vi "MainV1.vi"() -> ()   [LabVIEW 2019]
uses:
  <vilib>/userDefined/High Color/IMAQdx.ctl
  <vilib>/FPGAPlugInAG/myRIO-1900/niLvFpga_Open_myRIO-1900.vi
  <vilib>/rvi/interface/common/dynamic/niFpgaDynamicAddResources.vi
  <vilib>/Utility/error.llb/Error Cluster From Error Code.vi
  <vilib>/rvi/errors/niLvFpgaAdjustHostInterfaceError.vi
  <vilib>/FPGAPlugInAG/Dynamic/niLvFpga_Close_Dynamic.vi
  <vilib>/rvi/interface/nirviOpenFPGA/nirviOpenFPGA.xnode
  FPGA Bitfiles/MRmecanum_FPGATarget_FPGAMainModified_TerasRobot_LKSN2021.lvbitx
  <vilib>/rvi/interface/nirviReadWriteControl/nirviReadWriteControl.xnode
  <vilib>/rvi/interface/nirviCloseFPGA/nirviCloseFPGA.xnode
  NiFpgaLv.dll
  <vilib>/rvi/interface/Simulation/niFpgaSimulationCallBeginRW.vi
  <vilib>/vision/driver/NI_Vision_Acquisition_Software.lvlib
  <vilib>/vision/NI_Vision_Development_Module.lvlib
panel:
  out "Color Put":T1(plugin-control)
  in  "SERVO 3":u16
  in  "Value diatas brp?":u16
  in  "Value Udah ambil brp?":u16
  in  "M5  DOWN TIMES GRAB":u32=1
  in  "Udah ambil brp?":u16
  in  "Standcube diatas brp?":u16
  out "WHITE":bool
  out "TOXIC":bool
  out "BLUE":bool
  out "STOP ? 11":bool
  out "STOP ? 10":bool
  out "STOP ? 9":bool
  out "STOP ? 8":bool
  out "M5 up":i16=1000
  out "STOP ? 7":bool
  out "STOP ? 6":bool
  out "STOP ? 5":bool
  out "STOP ? 4":bool
  out "STOP ? 3":bool
  out "AND green":bool
  out "AND red":bool
  out "Red True":bool
  out "Green True":bool
  out "Locate Put":string
  out "Green Stand":bool
  out "Red Stand":bool
  out "STOP Open Grab":bool
  out "total":i16
  out "Index ke?":i32
  out "White Cube":bool
  out "Blue Cube":bool
  out "Toxic Cube":bool
  out "Color Grab":T1(plugin-control)
  in  "Color Sensitivity":u32(ring) items=["Low", "Medium", "High"]
  in  "Exposure Config Value":i64=10
  out "size(s)":i32
  in  "Session In":T2="cam1"
  out "Qrcode image":T1(plugin-control)
  out "Found ?":bool
  in  "Tab Control":T3(tab)
  in  "Main":T4(array[cluster])=[{"Time"=0.0, "Mode"=enum."Balance", "Speed"=250.0, "Gerakan"=enum."Maju"}, {"Time"=0.0, "Mode"=enum."Line Follow", "Speed"=150.0, "Gerakan"=enum."Kanan"}, {"Time"=0.0, "Mode"=enum."Qrcode", "Speed"=0.0, "Gerakan"=enum."Camera"}, {"Time"=1000.0, "Mode"=enum."Standard", "Speed"=100.0, "Gerakan"=enum."Mundur"}, {"Time"=3000.0, "Mode"=enum."Standard", "Speed"=300.0, "Gerakan"=enum."Kiri"}, {"Time"=0.0, "Mode"=enum."Balance", "Speed"=300.0, "Gerakan"=enum."Maju"}, {"Time"=2000.0, "Mode"=enum."Standard", "Speed"=815.0, "Gerakan"=enum."Putar Kiri"}, {"Time"=1300.0, "Mode"=enum."Standard", "Speed"=300.0, "Gerakan"=enum."Maju"}, {"Time"=0.0, "Mode"=enum."Balance", "Speed"=300.0, "Gerakan"=enum."Kanan"}, {"Time"=2100.0, "Mode"=enum."Standard", "Speed"=300.0, "Gerakan"=enum."Kiri"}]
  in  "Nurse":T4(array[cluster])=[{"Time"=2.0, "Mode"=enum."Standard", "Speed"=815.0, "Gerakan"=enum."Putar Kiri"}, {"Time"=0.0, "Mode"=enum."Balance", "Speed"=150.0, "Gerakan"=enum."Kiri"}, {"Time"=4.0, "Mode"=enum."Standard", "Speed"=300.0, "Gerakan"=enum."Maju"}, {"Time"=0.0, "Mode"=enum."Balance", "Speed"=150.0, "Gerakan"=enum."Kiri"}, {"Time"=0.0, "Mode"=enum."Line Follow", "Speed"=150.0, "Gerakan"=enum."Kanan"}, {"Time"=0.0, "Mode"=enum."Color Grab", "Speed"=0.0, "Gerakan"=enum."Camera"}, {"Time"=0.0, "Mode"=enum."Line Follow", "Speed"=200.0, "Gerakan"=enum."Kanan"}, {"Time"=0.0, "Mode"=enum."Color Put", "Speed"=0.0, "Gerakan"=enum."Camera"}]
  in  "Room 1":T4(array[cluster])
  in  "Room 2":T4(array[cluster])
  in  "Output":T4(array[cluster])=[{"Time"=0.0, "Mode"=enum."Balance", "Speed"=150.0, "Gerakan"=enum."Mundur"}, {"Time"=0.0, "Mode"=enum."Balance", "Speed"=150.0, "Gerakan"=enum."Kiri"}, {"Time"=5.0, "Mode"=enum."Standard", "Speed"=350.0, "Gerakan"=enum."Kanan"}, {"Time"=1.5, "Mode"=enum."Standard", "Speed"=1075.0, "Gerakan"=enum."Putar Kanan"}, {"Time"=0.0, "Mode"=enum."Balance", "Speed"=200.0, "Gerakan"=enum."Kanan"}, {"Time"=0.0, "Mode"=enum."Line Follow", "Speed"=200.0, "Gerakan"=enum."Kiri"}, {"Time"=1.5, "Mode"=enum."Standard", "Speed"=1075.0, "Gerakan"=enum."Putar Kiri"}, {"Time"=0.0, "Mode"=enum."Balance", "Speed"=300.0, "Gerakan"=enum."Kiri"}, {"Time"=0.0, "Mode"=enum."Balance", "Speed"=150.0, "Gerakan"=enum."Mundur"}]
  in  "Go Nurse":T4(array[cluster])
  in  "Go Room 1":T4(array[cluster])
  in  "Go Room 2":T4(array[cluster])
  out "Gerakan":T5(ring)
  out "Data":string
  out "Speed":dbl
  out "TIME":u32
  out "Splitted":string[](array[string])
  out "Mode":T6(ring)
  in  "error in":errorcluster
  out "error out":errorcluster
  out "M5 down":i16=1000
  out "* times":dbl
  in  "Gripper Close":u16=2900
  in  "Gripper Open":u16=3369
  in  "Servo 2 (centering)":u16=5630
  in  "Velocity Y Grab":dbl[](array[numeric])=[0.0, 0.0, 0.0]
  in  "Time Velocity Y Grab":u32=800
  out "STOP Close Grab":bool
  out "toxic index true?":bool
  out "white index true?":bool
  out "blue index true?":bool
  out "Take BLUE":bool
  out "Take TOXIC":bool
  out "Take WHITE":bool
  out "GO RED":bool
  out "GO GREEN":bool
  in  "Servo 2 (color detection stand cube)":u16=5955
  in  "M5  DOWN TIMES PUT":u32=1
  in  "Stop":bool
  # "DAVE"
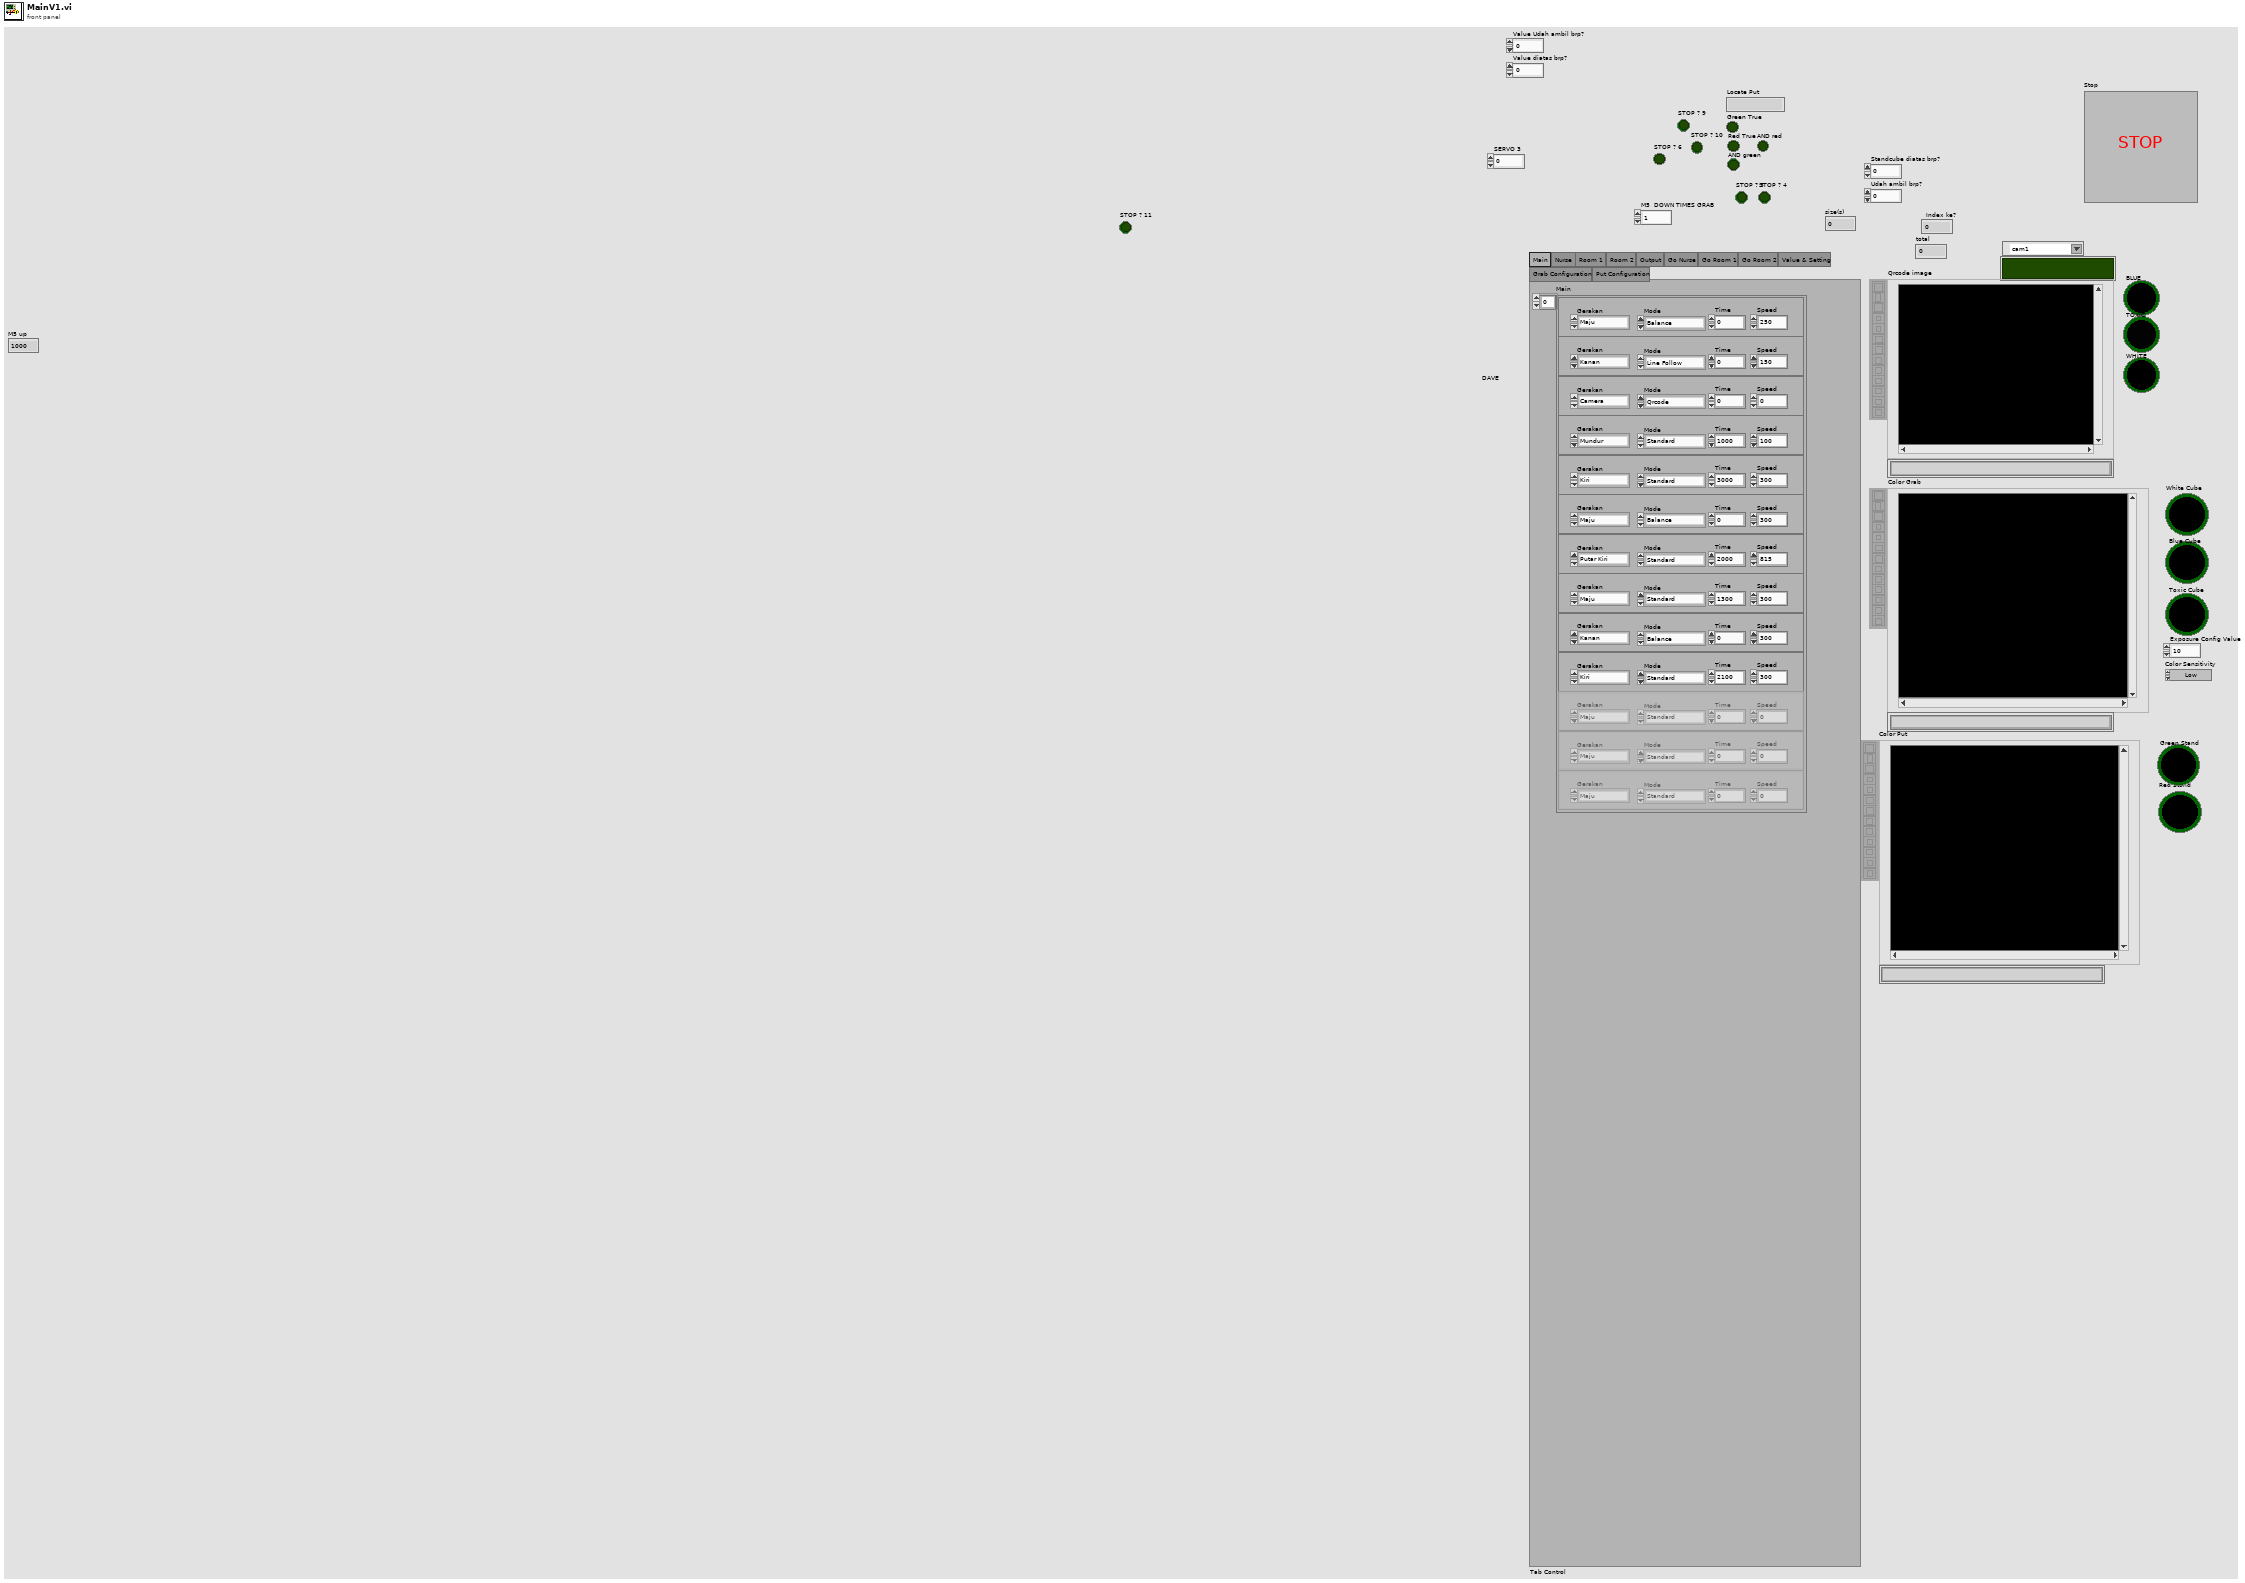
[diagram p1: front panel]
types:
  T1 = typedef "IMAQ Image.ctl" = refnum<image>
  T2 = typedef "IMAQdx.ctl" = refnum<k21>
  T3 = enum32{"Main", "Nurse", "Room 1", "Room 2", "Output", "Go Nurse", "Go Room 1", "Go Room 2", "Value & Setting", "Grab Configuration", "Put Configuration"}
  T4 = cluster{"Time":dbl, "Mode":enum16{"Standard", "Balance", "Line Follow", "Qrcode", "Color Grab", "Color Put", "GoNurse", "Go1", "Go2"}, "Speed":dbl, "Gerakan":enum16{"Maju", "Mundur", "Kiri", "Kanan", "Putar Kiri", "Putar Kanan", "Camera"}}[]
  T5 = enum16{"Maju", "Mundur", "Kiri", "Kanan", "Putar Kiri", "Putar Kanan", "Camera"}
  T6 = enum16{"Standard", "Balance", "Line Follow", "Qrcode", "Color Grab", "Color Put", "GoNurse", "Go1", "Go2"}
  T7 = enum16{"color detection", "grab", "down", "stop"}
  T8 = enum16{"color detection", "nurse", "room", "false", "true", "stop"}
  T9 = cluster{"Time":dbl, "Mode":enum16{"Standard", "Balance", "Line Follow", "Qrcode", "Color Grab", "Color Put", "GoNurse", "Go1", "Go2"}, "Speed":dbl, "Gerakan":enum16{"Maju", "Mundur", "Kiri", "Kanan", "Putar Kiri", "Putar Kanan", "Camera"}}
  T10 = typedef "Image Type" = u32
  T11 = typedef "QR Code Report.ctl" = cluster{"Found?":bool, "Data":string, "Bounding Box":cluster{"x":sgl, "y":sgl}[], "Errors Corrected":u32, "Dimensions (Rows/Cols)":u32, "Version":u32, "QR Model":T12, "Stream Mode":T13, "Barcode Polarity":T14, "Mirrored?":bool, "Append Stream Position":u32, "Size of Append Stream":u32, "First EAN-128 ID":i32, "First Alternate Language ID":i32, "Append Stream ID":u32, "Minimum Edge Strength":u32, "Demodulation Mode":T15, "Cell Sample Size":T16, "Cell Filter Mode":T17}
  T12 = typedef "QR Code Model Type.ctl" = i32
  T13 = typedef "QR Code Stream Mode Type.ctl" = i32
  T14 = typedef "Data Matrix Polarity.ctl" = i32
  T15 = typedef "Demodulation Mode.ctl" = i32
  T16 = typedef "Cell Sample Size.ctl" = i32
  T17 = typedef "Cell Filter Mode.ctl" = i32
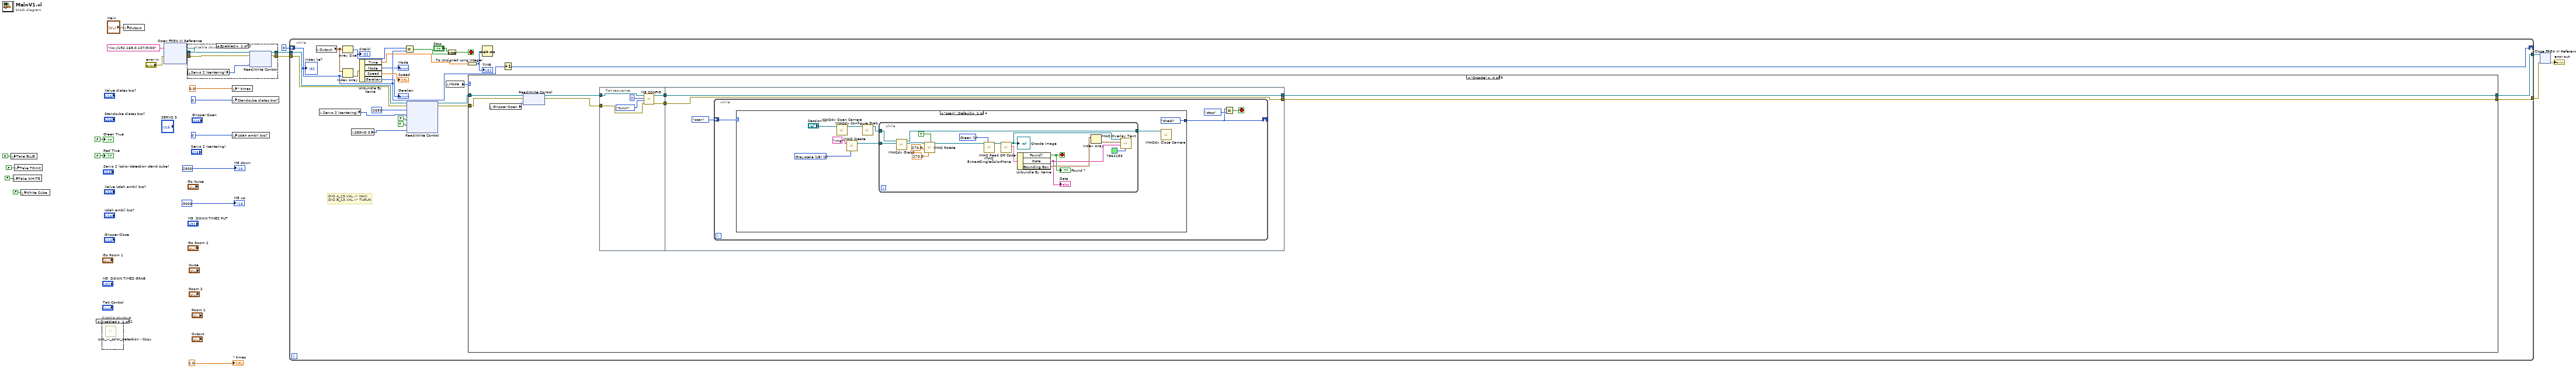
[diagram p0: block diagram]
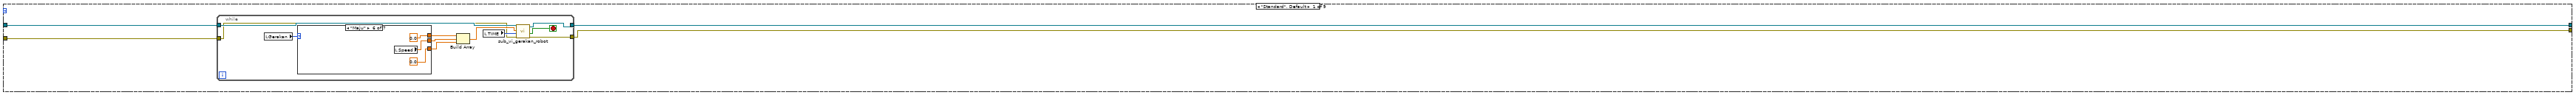
[diagram p4: hidden frame]
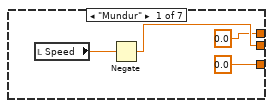
[diagram p5: hidden frame]
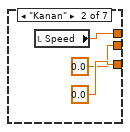
[diagram p6: hidden frame]
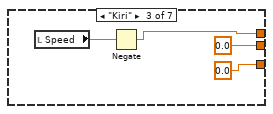
[diagram p7: hidden frame]
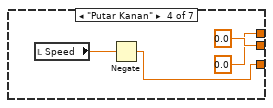
[diagram p8: hidden frame]
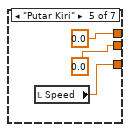
[diagram p9: hidden frame]
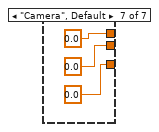
[diagram p10: hidden frame]
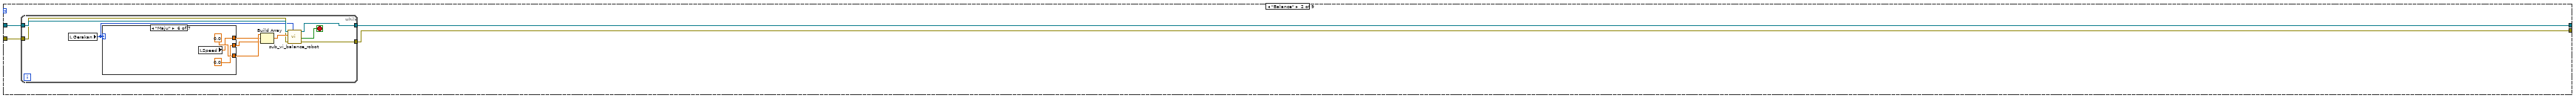
[diagram p11: hidden frame]
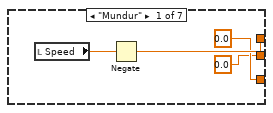
[diagram p12: hidden frame]
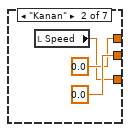
[diagram p13: hidden frame]
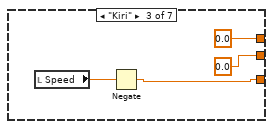
[diagram p14: hidden frame]
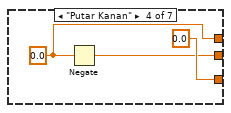
[diagram p15: hidden frame]
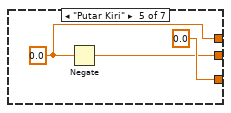
[diagram p16: hidden frame]
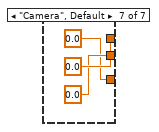
[diagram p17: hidden frame]
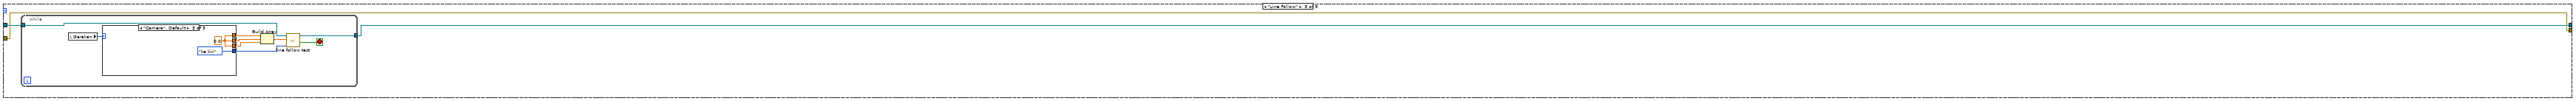
[diagram p18: hidden frame]
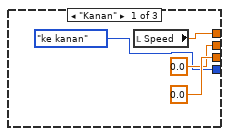
[diagram p19: hidden frame]
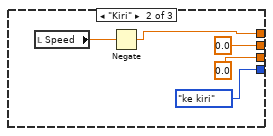
[diagram p20: hidden frame]
diagram:
  n1 = local write "Take BLUE"(FALSE ("Take BLUE")) -> ()
  n2 = local write "Take WHITE"(FALSE ("Take WHITE")) -> ()
  n3 = local write "Take TOXIC"(FALSE ("Take TOXIC")) -> ()
  n4 = local write "White Cube"(FALSE ("White Cube")) -> ()
  n5 = disable-structure shown="Disabled" {
    frame Disabled {
      n6 = call "sub_vi_color_detection - Copy.vi"() -> ()  [unwired: 8 in, 4 out]
    }
    frame Enabled {
    }
  }
  n7 = local write "Output"("Main") -> ()
  n8 = xnode "Open FPGA VI Reference"("error in"="error in", "resource name"=tag "rio://192.168.0.107/RIO0") -> ("FPGA VI Reference Out"=w22:refnum<k20>, "error out"=w11:errorcluster)
  n9 = disable-structure shown="Enabled" {
    disable-tunnel: w22 -> [w28 w30]
    disable-tunnel: [w27 w30] -> w12
    disable-tunnel: w11 -> [w26 w29]
    disable-tunnel: [w25 w29] -> w10
    frame Enabled {
      n10 = local read "Servo 2 (centering)"() -> (w24:u16)
      n11 = xnode "Read/Write Control"("FPGA VI Reference In"=w28, "error in"=w26, "SERVO 2"=w24) -> ("FPGA VI Reference Out"=w27:refnum<k20>, "error out"=w25:errorcluster)  [unwired: 1 in]
    }
    frame Disabled {
    }
  }
  n12 = local write "* times"(0.0 ("* times")) -> ()
  n13 = local write "Standcube diatas brp?"(u16 0 ("Standcube diatas brp?")) -> ()
  n14 = local write "Udah ambil brp?"(u16 0 ("Udah ambil brp?")) -> ()
  n15 = while {
    tunnel: w12 -> [w55]
    tunnel: [w48] -> w23
    shift-right: [w54] -> _
    shift-left: 0 -> [w49]
    tunnel: w10 -> [w41]
    tunnel: [w40] -> w17
    stop <- w46 stop-if-true
    # "DIO.A_13.VAL -> NAIK \nDIO.B_13.VAL -> TURUN"
    n16 = local read "Output"() -> (w51:T4)
    n17 = local read "Servo 2 (centering)"() -> (w32:u16)
    n18 = Array Size(array=w51) -> (size(s)=w50:i32)
    "size(s)" <- w50
    n19 = Index Array(array=w51, index=w49) -> (element=w53:T9)
    n20 = local read "SERVO 3"() -> (w33:u16)
    n21 = Unbundle By Name(w53) -> ("Time"=w31:dbl, "Mode"=→"Mode":T6, "Speed"=→"Speed":dbl, "Gerakan"=→"Gerakan":T5)
    n22 = Equal?(x=w50, y=w49) -> (x = y?=w47:bool)
    n23 = xnode "Read/Write Control"("FPGA VI Reference In"=w55, "error in"=w41, "M5"=i16 2650, "SERVO 2"=w32, "DIO.B_13.VAL"=FALSE, "DIO.A_13.VAL"=TRUE, "SERVO 3"=w33) -> ("FPGA VI Reference Out"=w38:refnum<k20>, "error out"=w37:errorcluster)
    n24 = local read "Mode"() -> (w43:T6)
    n25 = Exclusive Or(1:w47, 2:"Stop") -> (0:w46:bool)
    n26 = To Unsigned Long Integer(number=w31) -> (unsigned 32bit integer=w42:u32)
    "TIME" <- w42
    n27 = case shown="\"Qrcode\"" w43 {
      tunnel: w38 -> [w59 w98 w134 w162 w241 w487 w877 w893 w909]
      tunnel: [w58 w97 w133 w159 w237 w483 w875 w891 w907] -> w48
      tunnel: w37 -> [w57 w96 w132 w157 w239 w486 w876 w892 w908]
      tunnel: [w56 w95 w132 w163 w235 w484 w874 w890 w906] -> w40
      frame "Standard", Default {
        n28 = while {
          tunnel: w59 -> [w63]
          tunnel: [w62] -> w58
          tunnel: w57 -> [w61]
          tunnel: [w60] -> w56
          stop <- w65 stop-if-true
          n29 = local read "Gerakan"() -> (w70:T5)
          n30 = case shown="\"Maju\"" w70 {
            tunnel: [0.0 ("element") w76 w79 0.0 ("element") 0.0 ("element") 0.0 ("element") 0.0 ("element")] -> w69
            tunnel: [0.0 ("element") 0.0 ("element") 0.0 ("element") w82 w87 0.0 ("element") 0.0 ("element")] -> w68
            tunnel: [w73 0.0 ("element") 0.0 ("element") 0.0 ("element") 0.0 ("element") w89 0.0 ("element")] -> w67
            frame "Mundur" {
              n31 = local read "Speed"() -> (w74:dbl)
              n32 = Negate(x=w74) -> (-x=w73:dbl)
            }
            frame "Kanan" {
              n33 = local read "Speed"() -> (w76:dbl)
            }
            frame "Kiri" {
              n34 = local read "Speed"() -> (w80:dbl)
              n35 = Negate(x=w80) -> (-x=w79:dbl)
            }
            frame "Putar Kanan" {
              n36 = local read "Speed"() -> (w84:dbl)
              n37 = Negate(x=w84) -> (-x=w82:dbl)
            }
            frame "Putar Kiri" {
              n38 = local read "Speed"() -> (w87:dbl)
            }
            frame "Maju" {
              n39 = local read "Speed"() -> (w89:dbl)
            }
            frame "Camera", Default {
            }
          }
          n40 = Build Array(w69, w67, w68) -> (w66:dbl[])
          n41 = local read "TIME"() -> (w64:u32)
          n42 = call "sub_vi_gerakan_robot.vi"("error out"=w61, "Numeric"=w64, "steering frame velocity"=w66, "FPGA VI Reference Out"=w63) -> ("error out 2"=w60:errorcluster, "STOP ?"=w65:bool, "FPGA VI Reference Out 2"=w62:refnum<k20>)  [unwired: 5 in]
        }
      }
      frame "Balance" {
        n43 = while {
          tunnel: w98 -> [w104]
          tunnel: [w103] -> w97
          tunnel: w96 -> [w100]
          tunnel: [w99] -> w95
          stop <- w105 stop-if-true
          n44 = local read "Gerakan"() -> (w102:T5)
          n45 = case shown="\"Maju\"" w102 {
            tunnel: [0.0 ("element") w113 w116 0.0 ("element") 0.0 ("element") 0.0 ("element") 0.0 ("element")] -> w108
            tunnel: [0.0 ("element") 0.0 ("element") 0.0 ("element") w121 w124 0.0 ("element") 0.0 ("element")] -> w101
            tunnel: [w111 0.0 ("element") 0.0 ("element") w120 w123 w126 0.0 ("element")] -> w107
            frame "Mundur" {
              n46 = local read "Speed"() -> (w112:dbl)
              n47 = Negate(x=w112) -> (-x=w111:dbl)
            }
            frame "Kanan" {
              n48 = local read "Speed"() -> (w113:dbl)
            }
            frame "Kiri" {
              n49 = local read "Speed"() -> (w118:dbl)
              n50 = Negate(x=w118) -> (-x=w116:dbl)
            }
            frame "Putar Kanan" {
              w120 = 0.0 ("element")
              n51 = Negate(x=w120) -> (-x=w121:dbl)
            }
            frame "Putar Kiri" {
              w123 = 0.0 ("element")
              n52 = Negate(x=w123) -> (-x=w124:dbl)
            }
            frame "Maju" {
              n53 = local read "Speed"() -> (w126:dbl)
            }
            frame "Camera", Default {
            }
          }
          n54 = Build Array(w108, w107, w101) -> (w106:dbl[])
          n55 = call "sub_vi_balance_robot.vi"("Gerakan"=w102, "error out"=w100, "steering frame velocity"=w106, "FPGA VI Reference Out"=w104) -> ("error out 2"=w99:errorcluster, "Stop ?"=w105:bool, "FPGA VI Reference Out 2"=w103:refnum<k20>)  [unwired: 5 in]
        }
      }
      frame "Line Follow" {
        n56 = while {
          tunnel: w134 -> [w138]
          tunnel: [w137] -> w133
          stop <- w136 stop-if-true
          n57 = local read "Gerakan"() -> (w143:T5)
          n58 = case shown="\"Camera\", Default" w143 {
            tunnel: [w144 w148 w153] -> w142
            tunnel: [0.0 ("element") 0.0 ("element") w153] -> w141
            tunnel: [0.0 ("element") 0.0 ("element") w153] -> w140
            tunnel: [enum16{"ke kiri", "ke kanan"}."ke kanan" ("Options") enum16{"ke kiri", "ke kanan"}."ke kiri" ("Options") enum16{"ke kiri", "ke kanan"}."ke kiri" ("Options")] -> w135
            frame "Kanan" {
              n59 = local read "Speed"() -> (w144:dbl)
            }
            frame "Kiri" {
              n60 = local read "Speed"() -> (w149:dbl)
              n61 = Negate(x=w149) -> (-x=w148:dbl)
            }
            frame "Camera", Default {
              w153 = 0.0 ("element")
            }
          }
          n62 = Build Array(w142, w140, w141) -> (w139:dbl[])
          n63 = call "line follow test.vi"("FPGA VI Reference Out"=w138, "steering frame velocity"=w139, "Options"=w135) -> ("FPGA VI Reference Out 2"=w137:refnum<k20>, "STOP ?"=w136:bool)  [unwired: 6 in]
        }
      }
      frame "Qrcode" {
        n64 = local read "Gripper Open"() -> (w155:u16)
        n65 = xnode "Read/Write Control"("FPGA VI Reference In"=w162, "error in"=w157, "SERVO 3"=w155) -> ("FPGA VI Reference Out"=w158:refnum<k20>, "error out"=w156:errorcluster)
        n66 = flat-sequence {
          tunnel: w158 -> [w165]
          tunnel: w156 -> [w169]
          tunnel: [w168] -> w161
          tunnel: [w164] -> w160
          tunnel: [w171] -> w163
          tunnel: w161 -> [w171]
          tunnel: [w170] -> w159
          tunnel: w160 -> [w170]
          frame #0 {
            n67 = call "M5 CONFIG.vi"("error in"=w169, "Enum"=enum16{"naik", "turun"}."turun", "berapa kali?"=u32 2, "FPGA VI Reference Out"=w165) -> ("error out"=w168:errorcluster, "FPGA VI Reference Out 2"=w164:refnum<k20>)  [unwired: 6 in]
          }
          frame #1 {
            n68 = while {
              shift-right: [w174] -> _
              shift-left: enum16{"scan", "check", "insert", "stop"}."scan" -> [w176]
              stop <- w173 stop-if-true
              n69 = case shown="\"scan\", Default" w176 {
                tunnel: [enum16{"scan", "check", "insert", "stop"}."check" enum16{"scan", "check", "insert", "stop"}."insert" enum16{"scan", "check", "insert", "stop"}."stop" enum16{"scan", "check", "insert", "stop"}."stop"] -> w174
                frame "scan", Default {
                  w181 = T10 0 items=["Grayscale (U8)", "Grayscale (I16)", "Grayscale (SGL)", "Complex (CSG)", "RGB (U32)", "HSL (U32)", "RGB (U64)", "Grayscale (U16)"] ("Image Type")
                  n70 = call <vilib>:"IMAQdx Open Camera.vi"("Session In"="Session In") -> ("Session Out"=w183:T2)  [unwired: 9 in, 1 out]
                  n71 = call "IMAQ Create"("Image Name"="img", "Image Type"=w181) -> ("New Image"=w180:T1)  [unwired: 3 in, 1 out]
                  n72 = call <vilib>:"IMAQdx Configure Grab.vi"("Session In"=w183) -> ("Session Out"=w182:T2)  [unwired: 9 in, 1 out]
                  n73 = while {
                    tunnel: w182 -> [w201]
                    tunnel: w180 -> [w200]
                    tunnel: [w190] -> w177
                    stop <- w196 stop-if-true
                    w199 = 1 items=["Red", "Green", "Blue", "Hue", "Saturation", "Luminance", "Value", "Intensity"] ("Color Plane")
                    n74 = call <vilib>:"IMAQdx Grab2.vi"("Image In"=w200, "Session In"=w201) -> ("Image Out"=w189:T1, "Session Out"=w190:T2)  [unwired: 6 in, 2 out]
                    n75 = call "IMAQ Rotate"("Maintain Size"=TRUE, "Replace Value"=sgl 270.0, "Angle (degrees)"=sgl 270.0, "Image Src"=w189) -> ("Image Dst Out"=w188:T1)  [unwired: 6 in, 1 out]
                    n76 = call "IMAQ ExtractSingleColorPlane"("Color Plane"=w199, "Image Src"=w188) -> ("Image Dst Out"=w198:T1)  [unwired: 8 in, 1 out]
                    n77 = call "IMAQ Read QR Code"("Image"=w198) -> ("QR Code Report"=w197:T11, "Image (duplicate)"=w191:T1)  [unwired: 7 in, 2 out]
                    "Qrcode image" <- w191
                    n78 = Unbundle By Name(w197) -> ("Found?"=w196:bool, "Data"=w193:string, "Bounding Box"=w195:cluster{"x":sgl, "y":sgl}[])
                    "Found ?" <- w196
                    "Data" <- w193
                    n79 = Index Array(array=w195) -> (element=w194:cluster{"x":sgl, "y":sgl})  [unwired: 1 in]
                    n80 = call "IMAQ Overlay Text"("Text Color (black)"=u32 7864153, "String"=w193, "Origin"=w194, "Image"=w191) -> ()  [unwired: 6 in, 2 out]
                  }
                  n81 = call <vilib>:"IMAQdx Close Camera.vi"("Session In"=w177) -> ()  [unwired: 10 in, 1 out]
                }
                frame "check" {
                  n82 = local read "Data"() -> (w202:string)
                  n83 = call "SplitStringToArray SubVI.vi"("String"=w202) -> ("Array"=→"Splitted":string[])  [unwired: 10 in]
                }
                frame "insert" {
                  w208 = "1" ("y")
                  n84 = local read "Splitted"() -> (w215:string[])
                  n85 = local read "Splitted"() -> (w219:string[])
                  n86 = Index Array(array=w219, index=1) -> (element=w218:string)
                  "Locate Put" <- w218
                  n87 = Index Array(array=w215, index #1=7 ("index"), index #2=8 ("index"), index #3=9 ("index")) -> (element #1=w211:string, element #2=w210:string, element #3=w209:string)
                  n88 = Equal?(x=w211, y=w208) -> (x = y?=→"BLUE":bool)
                  n89 = Equal?(x=w210, y=w208) -> (x = y?=→"TOXIC":bool)
                  n90 = Equal?(x=w209, y=w208) -> (x = y?=→"WHITE":bool)
                  n91 = case shown="\"N\", Default" w218 {
                    frame "N", Default {
                      n92 = local read "Output"() -> (w221:T4)
                      n93 = local read "size(s)"() -> (w222:i32)
                      n94 = local read "Nurse"() -> (w223:T4)
                      n95 = Insert Into Array(array=w221, index=w222, new element=w223) -> (w220:T4)
                      n96 = local write "Output"(w220) -> ()
                    }
                    frame "1" {
                      n97 = local read "Room 1"() -> (w227:T4)
                      n98 = local read "Output"() -> (w225:T4)
                      n99 = local read "size(s)"() -> (w226:i32)
                      n100 = Insert Into Array(array=w225, index=w226, new element=w227) -> (w224:T4)
                      n101 = local write "Output"(w224) -> ()
                    }
                    frame "2" {
                      n102 = local read "Room 2"() -> (w231:T4)
                      n103 = local read "Output"() -> (w229:T4)
                      n104 = local read "size(s)"() -> (w230:i32)
                      n105 = Insert Into Array(array=w229, index=w230, new element=w231) -> (w228:T4)
                      n106 = local write "Output"(w228) -> ()
                    }
                  }
                }
                frame "stop" {
                }
              }
              n107 = Equal?(x=w174, y=enum16{"scan", "check", "insert", "stop"}."stop") -> (x = y?=w173:bool)
            }
          }
        }
      }
      frame "Color Grab" {
        n108 = local read "Splitted"() -> (w257:string[])
        n109 = local read "Splitted"() -> (w258:string[])
        n110 = local read "Udah ambil brp?"() -> (w233:u16)
        n111 = local read "Splitted"() -> (w259:string[])
        n112 = Index Array(array=w257, index=7) -> (element=w251:string)
        n113 = Index Array(array=w258, index=8) -> (element=w260:string)
        n114 = case shown="2" w233 {
          frame 1 {
            n115 = local write "Value Udah ambil brp?"(u16 2 ("Value Udah ambil brp?")) -> ()
          }
          frame 0, Default {
            n116 = local write "Value Udah ambil brp?"(u16 0 ("Value Udah ambil brp?")) -> ()
          }
          frame 2 {
            n117 = local write "Value Udah ambil brp?"(u16 4 ("Value Udah ambil brp?")) -> ()
          }
        }
        n118 = while {
          shift-right: [w266] -> _
          shift-left: T7."color detection" -> [w269]
          tunnel: w241 -> [w271]
          tunnel: [w270] -> w238
          tunnel: [w268] -> w236
          tunnel: w239 -> [w265]
          stop <- w272 stop-if-true
          n119 = case shown="\"grab\"" w269 {
            tunnel: w271 -> [w289 w340 w412 w473]
            tunnel: [w283 w342 w407 w473] -> w270
            tunnel: [w284 w341 w408 w472] -> w268
            tunnel: [w282 w338 w410 T7."stop"] -> w266
            tunnel: w265 -> [w281 w336 w406 w472]
            frame "grab" {
              n120 = flat-sequence {
                tunnel: w281 -> [w295]
                tunnel: w289 -> [w291]
                tunnel: [w294] -> w280
                tunnel: [w290] -> w278
                tunnel: w280 -> [w298]
                tunnel: [w296] -> w279
                tunnel: w278 -> [w299]
                tunnel: [w297] -> w277
                tunnel: [w316] -> w288
                tunnel: [w315] -> w287
                tunnel: w279 -> [w312]
                tunnel: w277 -> [w310]
                tunnel: w288 -> [w320]
                tunnel: w287 -> [w321]
                tunnel: [w319] -> w286
                tunnel: [w318] -> w285
                tunnel: w286 -> [w329]
                tunnel: w285 -> [w328]
                tunnel: [w323] -> w276
                tunnel: [w322] -> w274
                tunnel: w276 -> [w332]
                tunnel: [w332] -> w275
                tunnel: w274 -> [w331]
                tunnel: [w331] -> w273
                tunnel: [w333] -> w283
                tunnel: [w334] -> w284
                tunnel: [T7."stop"] -> w282
                tunnel: w275 -> [w334]
                tunnel: w273 -> [w333]
                frame #0 {
                  n121 = call "M5 CONFIG.vi"("error in"=w295, "Enum"=enum16{"naik", "turun"}."turun", "berapa kali?"=u32 0, "FPGA VI Reference Out"=w291) -> ("error out"=w294:errorcluster, "FPGA VI Reference Out 2"=w290:refnum<k20>)  [unwired: 6 in]
                }
                frame #1 {
                  n122 = local read "Udah ambil brp?"() -> (w302:u16)
                  n123 = Equal?(x=w302, y=u16 2) -> (x = y?=w300:bool)
                  n124 = case shown="True" w300 {
                    tunnel: w299 -> [w304 w309]
                    tunnel: w298 -> [w303 w308]
                    tunnel: [w304 w307] -> w297
                    tunnel: [w303 w306] -> w296
                    frame False {
                    }
                    frame True {
                      n125 = xnode "Read/Write Control"("FPGA VI Reference In"=w309, "error in"=w308, "SERVO 3"=u16 5920) -> ("FPGA VI Reference Out"=w307:refnum<k20>, "error out"=w306:errorcluster)
                    }
                  }
                }
                frame #2 {
                  n126 = call "sub_vi_gerakan_robot.vi"("error out"=w312, "Numeric"="Time Velocity Y Grab", "steering frame velocity"="Velocity Y Grab", "FPGA VI Reference Out"=w310) -> ("error out 2"=w316:errorcluster, "STOP ?"=→"STOP Open Grab":bool, "FPGA VI Reference Out 2"=w315:refnum<k20>)  [unwired: 5 in]
                }
                frame #3 {
                  n127 = xnode "Read/Write Control"("FPGA VI Reference In"=w321, "error in"=w320, "SERVO 3"=u16 2824) -> ("FPGA VI Reference Out"=w319:refnum<k20>, "error out"=w318:errorcluster)
                }
                frame #4 {
                  n128 = local read "Velocity Y Grab"() -> (w327:dbl[])
                  n129 = local read "Time Velocity Y Grab"() -> (w325:u32)
                  n130 = Negate(x=w327) -> (-x=w326:dbl[])
                  n131 = call "sub_vi_gerakan_robot.vi"("error out"=w328, "Numeric"=w325, "steering frame velocity"=w326, "FPGA VI Reference Out"=w329) -> ("error out 2"=w323:errorcluster, "STOP ?"=→"STOP Close Grab":bool, "FPGA VI Reference Out 2"=w322:refnum<k20>)  [unwired: 5 in]
                }
                frame #5 {
                  n132 = local write "SERVO 3"(u16 2824 ("SERVO 3")) -> ()
                }
                frame #6 {
                }
              }
            }
            frame "down" {
              n133 = flat-sequence {
                tunnel: w340 -> [w344]
                tunnel: [w344] -> w339
                tunnel: [w343] -> w337
                tunnel: w336 -> [w343]
                tunnel: [w351] -> w342
                tunnel: [w350] -> w341
                tunnel: w339 -> [w349]
                tunnel: [w348] -> w338
                tunnel: w337 -> [w347]
                frame #0 {
                  n134 = local read "Udah ambil brp?"() -> (w346:u16)
                  n135 = Increment(x=w346) -> (x+1=w345:u16)
                  n136 = local write "Udah ambil brp?"(w345) -> ()
                }
                frame #1 {
                  n137 = disable-structure shown="Enabled" {
                    disable-tunnel: [w357 w384] -> w351
                    disable-tunnel: [w356 w382] -> w350
                    disable-tunnel: w349 -> [w354 w385]
                    disable-tunnel: [w353 w379] -> w348
                    disable-tunnel: w347 -> [w352 w383]
                    frame Disabled {
                      n138 = local read "* times"() -> (w358:dbl)
                      n139 = Greater?(x=w358, y=2.0) -> (0:w355:bool)
                      n140 = case shown="False" w355 {
                        tunnel: [w360 w378] -> w357
                        tunnel: [w366 w376] -> w356
                        tunnel: w354 -> [w364 w378]
                        tunnel: [w365 T7."stop"] -> w353
                        tunnel: w352 -> [w362 w376]
                        frame False {
                          n141 = flat-sequence {
                            tunnel: w364 -> [w368]
                            tunnel: [w372] -> w363
                            tunnel: w362 -> [w371]
                            tunnel: [w367] -> w361
                            tunnel: [w374] -> w366
                            tunnel: [T7."color detection"] -> w365
                            tunnel: w363 -> [w374]
                            tunnel: [w373] -> w360
                            tunnel: w361 -> [w373]
                            frame #0 {
                              n142 = call "M5 CONFIG.vi"("error in"=w371, "Enum"=enum16{"naik", "turun"}."turun", "berapa kali?"=u32 1, "FPGA VI Reference Out"=w368) -> ("error out"=w372:errorcluster, "FPGA VI Reference Out 2"=w367:refnum<k20>)  [unwired: 6 in]
                            }
                            frame #1 {
                            }
                          }
                        }
                        frame True {
                        }
                      }
                    }
                    frame Enabled {
                      n143 = flat-sequence {
                        tunnel: w385 -> [w389]
                        tunnel: w383 -> [w387]
                        tunnel: [w388] -> w381
                        tunnel: [w386] -> w380
                        tunnel: [w393] -> w382
                        tunnel: [w394] -> w384
                        tunnel: w381 -> [w394]
                        tunnel: w380 -> [w393]
                        tunnel: [T7."color detection"] -> w379
                        frame #0 {
                          n144 = call "M5 CONFIG.vi"("error in"=w387, "Enum"=enum16{"naik", "turun"}."turun", "berapa kali?"=u32 2, "FPGA VI Reference Out"=w389) -> ("error out"=w386:errorcluster, "FPGA VI Reference Out 2"=w388:refnum<k20>)  [unwired: 6 in]
                        }
                        frame #1 {
                        }
                      }
                    }
                  }
                }
              }
            }
            frame "color detection" {
              n145 = flat-sequence {
                tunnel: w406 -> [w414]
                tunnel: w412 -> [w417]
                tunnel: [w416] -> w398
                tunnel: [w415] -> w397
                tunnel: [w426] -> w405
                tunnel: w398 -> [w420]
                tunnel: w397 -> [w425]
                tunnel: [w419] -> w395
                tunnel: [w428] -> w400
                tunnel: w405 -> [w428]
                tunnel: [w427] -> w396
                tunnel: w395 -> [w427]
                tunnel: [w436] -> w401
                tunnel: w400 -> [w434]
                tunnel: [w435] -> w399
                tunnel: w396 -> [w433]
                tunnel: [w439] -> w411
                tunnel: [w438] -> w409
                tunnel: w401 -> [w440]
                tunnel: w399 -> [w437]
                tunnel: w411 -> [w461]
                tunnel: w409 -> [w448]
                tunnel: [w461] -> w404
                tunnel: [w449] -> w403
                tunnel: [w448] -> w402
                tunnel: [w469] -> w408
                tunnel: [w471] -> w410
                tunnel: [w467] -> w407
                tunnel: w404 -> [w468]
                tunnel: w403 -> [w471]
                tunnel: w402 -> [w470]
                frame #0 {
                  n146 = local read "Gripper Open"() -> (w413:u16)
                  n147 = xnode "Read/Write Control"("FPGA VI Reference In"=w417, "error in"=w414, "SERVO 3"=w413) -> ("FPGA VI Reference Out"=w416:refnum<k20>, "error out"=w415:errorcluster)
                }
                frame #1 {
                  n148 = local read "Value Udah ambil brp?"() -> (w422:u16)
                  n149 = To Unsigned Long Integer(number=w422) -> (unsigned 32bit integer=w421:u32)
                  n150 = Add(x=u32 0, y=w421) -> (x+y=w423:u32)
                  n151 = call "M5 CONFIG.vi"("error in"=w425, "Enum"=enum16{"naik", "turun"}."turun", "berapa kali?"=w423, "FPGA VI Reference Out"=w420) -> ("error out"=w426:errorcluster, "FPGA VI Reference Out 2"=w419:refnum<k20>)  [unwired: 6 in]
                }
                frame #2 {
                  n152 = local write "Take WHITE"(FALSE ("Take WHITE")) -> ()
                  n153 = local write "Take BLUE"(FALSE ("Take BLUE")) -> ()
                  n154 = local write "Take TOXIC"(FALSE ("Take TOXIC")) -> ()
                }
                frame #3 {
                  n155 = xnode "Read/Write Control"("FPGA VI Reference In"=w433, "error in"=w434, "SERVO 2"=u16 5390) -> ("FPGA VI Reference Out"=w436:refnum<k20>, "error out"=w435:errorcluster)
                }
                frame #4 {
                  # "BXW"
                  n156 = local read "Session In"() -> (w447:T2)
                  n157 = call "Color Detection new.vi"("error out"=w437, "Color Sensitivity"="Color Sensitivity", "Exposure Config Value"="Exposure Config Value", "Session In"=w447, "FPGA VI Reference Out"=w440) -> ("White Cube"=→"White Cube":bool, "Toxic Cube"=→"Toxic Cube":bool, "Blue Cube"=→"Blue Cube":bool, "FPGA VI Reference Out 2"=w439:refnum<k20>, "Image 2"=→"Color Grab":T1, "error out 2"=w438:errorcluster)  [unwired: 1 in]
                }
                frame #5 {
                  n158 = local read "white index true?"() -> (w455:bool)
                  n159 = local read "toxic index true?"() -> (w454:bool)
                  n160 = local read "White Cube"() -> (w452:bool)
                  n161 = local read "Toxic Cube"() -> (w451:bool)
                  n162 = local read "blue index true?"() -> (w453:bool)
                  n163 = local read "Blue Cube"() -> (w450:bool)
                  n164 = And(x=w454, y=w451) -> (x .and. y?=w457:bool)
                  "Take TOXIC" <- w457
                  n165 = And(x=w455, y=w452) -> (x .and. y?=w456:bool)
                  "Take WHITE" <- w456
                  n166 = Exclusive Or(1:w456, 2:w457) -> (0:w459:bool)
                  n167 = And(x=w453, y=w450) -> (x .and. y?=w458:bool)
                  "Take BLUE" <- w458
                  n168 = Exclusive Or(1:w459, 2:w458) -> (0:w460:bool)
                  n169 = case shown="False" w460 {
                    tunnel: [T7."down" T7."grab"] -> w449
                    frame False {
                    }
                    frame True {
                      n170 = local read "Udah ambil brp?"() -> (w463:u16)
                      n171 = Increment(x=w463) -> (x+1=w464:u16)
                      n172 = local write "Udah ambil brp?"(w464) -> ()
                    }
                  }
                }
                frame #6 {
                  n173 = xnode "Read/Write Control"("FPGA VI Reference In"=w468, "error in"=w470, "SERVO 2"=u16 5630) -> ("FPGA VI Reference Out"=w467:refnum<k20>, "error out"=w469:errorcluster)
                }
              }
            }
            frame "stop", Default {
            }
          }
          n174 = Equal?(x=w266, y=T7."stop") -> (x = y?=w272:bool)
        }
        n175 = Index Array(array=w259, index=9) -> (element=w261:string)
        n176 = Equal?(x=w251, y="1") -> (x = y?=w244:bool)
        "blue index true?" <- w244
        n177 = Equal?(x=w260, y="1") -> (x = y?=w243:bool)
        "toxic index true?" <- w243
        n178 = Boolean To (0,1)(Boolean=w244) -> (0, 1=w245:i16)
        n179 = Boolean To (0,1)(Boolean=w243) -> (0, 1=w246:i16)
        n180 = Equal?(x=w261, y="1") -> (x = y?=w242:bool)
        "white index true?" <- w242
        n181 = Add(x=w245, y=w246) -> (x+y=w248:i16)
        n182 = Boolean To (0,1)(Boolean=w242) -> (0, 1=w247:i16)
        n183 = Add(x=w248, y=w247) -> (x+y=→"total":i16)
        n184 = local read "Gripper Close"() -> (w234:u16)
        n185 = xnode "Read/Write Control"("FPGA VI Reference In"=w238, "error in"=w236, "SERVO 3"=w234) -> ("FPGA VI Reference Out"=w237:refnum<k20>, "error out"=w235:errorcluster)
      }
      frame "Color Put" {
        n186 = local read "Standcube diatas brp?"() -> (w475:u16)
        n187 = flat-sequence {
          tunnel: w486 -> [w491]
          tunnel: w487 -> [w494]
          tunnel: [w493] -> w479
          tunnel: [w492] -> w478
          tunnel: [w497] -> w482
          tunnel: [w496] -> w480
          tunnel: w479 -> [w499]
          tunnel: w478 -> [w498]
          tunnel: w482 -> [w504]
          tunnel: [w508] -> w481
          tunnel: w480 -> [w507]
          tunnel: [w505] -> w477
          tunnel: [w510] -> w485
          tunnel: w481 -> [w510]
          tunnel: w477 -> [w509]
          tunnel: [w509] -> w476
          tunnel: w485 -> [w529]
          tunnel: [w527] -> w484
          tunnel: [w526] -> w483
          tunnel: w476 -> [w525]
          frame #0 {
            n188 = local read "Gripper Close"() -> (w490:u16)
            n189 = xnode "Read/Write Control"("FPGA VI Reference In"=w494, "error in"=w491, "SERVO 3"=w490) -> ("FPGA VI Reference Out"=w493:refnum<k20>, "error out"=w492:errorcluster)
          }
          frame #1 {
            n190 = xnode "Read/Write Control"("FPGA VI Reference In"=w499, "error in"=w498, "SERVO 2"=u16 6500) -> ("FPGA VI Reference Out"=w497:refnum<k20>, "error out"=w496:errorcluster)
          }
          frame #2 {
            n191 = local read "Value diatas brp?"() -> (w502:u16)
            n192 = To Unsigned Long Integer(number=w502) -> (unsigned 32bit integer=w501:u32)
            n193 = Subtract(x=u32 2 ("berapa kali?"), y=w501) -> (x-y=w500:u32)
            n194 = call "M5 CONFIG.vi"("error in"=w507, "Enum"=enum16{"naik", "turun"}."turun", "berapa kali?"=w500, "FPGA VI Reference Out"=w504) -> ("error out"=w508:errorcluster, "FPGA VI Reference Out 2"=w505:refnum<k20>)  [unwired: 6 in]
          }
          frame #3 {
            n195 = local read "Take BLUE"() -> (w520:bool)
            n196 = local read "Take WHITE"() -> (w518:bool)
            n197 = Select(t="green", s=w520, f="") -> (s? t:f=w515:string)
            n198 = local read "Take TOXIC"() -> (w519:bool)
            n199 = Select(t="green", s=w518, f=w515) -> (s? t:f=w513:string)
            n200 = Select(t="red", s=w519, f=w513) -> (s? t:f=w511:string)
            n201 = case shown="\"red\"" w511 {
              frame "green", Default {
                n202 = local write "GO RED"(FALSE ("GO RED")) -> ()
                "GO GREEN" <- TRUE ("GO GREEN")
              }
              frame "red" {
                n203 = local write "GO GREEN"(FALSE ("GO GREEN")) -> ()
                "GO RED" <- TRUE ("GO RED")
              }
            }
          }
          frame #4 {
            n204 = while {
              tunnel: w529 -> [w537]
              shift-right: [w533] -> _
              shift-left: T8."color detection" -> [w534]
              tunnel: [w532] -> w527
              tunnel: [w531] -> w526
              tunnel: w525 -> [w530]
              stop <- w535 stop-if-true
              n205 = case shown="\"color detection\", Default" w534 {
                tunnel: w537 -> [w550 w589 w734 w763 w825 w873]
                tunnel: [w549 w587 w733 w755 w817 w871] -> w531
                tunnel: [w542 w584 w735 w756 w818 T8."stop"] -> w533
                tunnel: [w548 w588 w734 w754 w816 w873] -> w532
                tunnel: w530 -> [w546 w583 w733 w750 _ w871]
                frame "color detection", Default {
                  n206 = flat-sequence {
                    tunnel: [w554] -> w547
                    tunnel: [w551] -> w545
                    tunnel: w550 -> [w554]
                    tunnel: w546 -> [w551]
                    tunnel: w547 -> [w558]
                    tunnel: [w556] -> w541
                    tunnel: w545 -> [w559]
                    tunnel: [w557] -> w540
                    tunnel: w541 -> [w562]
                    tunnel: w540 -> [w565]
                    tunnel: [w564] -> w539
                    tunnel: [w563] -> w538
                    tunnel: w539 -> [w567]
                    tunnel: [w575] -> w544
                    tunnel: [w568] -> w543
                    tunnel: w538 -> [w574]
                    tunnel: [w578] -> w548
                    tunnel: [w579] -> w549
                    tunnel: w544 -> [w579]
                    tunnel: w543 -> [w578]
                    tunnel: [w576] -> w542
                    frame #0 {
                      n207 = local write "Green Stand"(FALSE ("Green Stand")) -> ()
                      n208 = local write "Red Stand"(FALSE ("Red Stand")) -> ()
                    }
                    frame #1 {
                      n209 = xnode "Read/Write Control"("FPGA VI Reference In"=w559, "error in"=w558, "SERVO 2"=u16 5630) -> ("FPGA VI Reference Out"=w557:refnum<k20>, "error out"=w556:errorcluster)
                    }
                    frame #2 {
                      n210 = call "M5 CONFIG.vi"("error in"=w562, "Enum"=enum16{"naik", "turun"}."turun", "berapa kali?"=u32 2, "FPGA VI Reference Out"=w565) -> ("error out"=w563:errorcluster, "FPGA VI Reference Out 2"=w564:refnum<k20>)  [unwired: 6 in]
                    }
                    frame #3 {
                      n211 = local read "Exposure Config Value"() -> (w573:i64)
                      n212 = local read "Color Sensitivity"() -> (w572:u32)
                      n213 = local read "Session In"() -> (w571:T2)
                      n214 = call "Color Detection Put.vi"("error out"=w574, "Color Sensitivity"=w572, "Exposure Config Value"=w573, "Session In"=w571, "FPGA VI Reference Out"=w567) -> ("Red Stand"=→"Red Stand":bool, "Green Stand"=→"Green Stand":bool, "FPGA VI Reference Out 2"=w575:refnum<k20>, "Image 2"=→"Color Put":T1, "error out 2"=w568:errorcluster)  [unwired: 2 in]
                    }
                    frame #4 {
                      n215 = local read "Locate Put"() -> (w577:string)
                      n216 = case shown="\"1\"" w577 {
                        tunnel: [T8."nurse" T8."room" T8."room"] -> w576
                        frame "N", Default {
                        }
                        frame "1" {
                        }
                        frame "2" {
                        }
                      }
                    }
                  }
                }
                frame "nurse" {
                  n217 = flat-sequence {
                    tunnel: w589 -> [w593]
                    tunnel: [w592] -> w586
                    tunnel: [w591] -> w585
                    tunnel: w583 -> [w590]
                    tunnel: [w731] -> w587
                    tunnel: [w732] -> w588
                    tunnel: w586 -> [w732]
                    tunnel: w585 -> [w731]
                    tunnel: [T8."stop"] -> w584
                    frame #0 {
                      n218 = while {
                        shift-right: [w601] -> _
                        shift-left: enum16{"check", "false", "true", "stop"}."check" -> [w602]
                        tunnel: w593 -> [w598]
                        tunnel: [w597] -> w592
                        tunnel: [w596] -> w591
                        tunnel: w590 -> [w595]
                        stop <- w599 stop-if-true
                        n219 = case shown="\"false\"" w602 {
                          tunnel: [w605 w626 enum16{"check", "false", "true", "stop"}."stop"] -> w601
                          tunnel: w598 -> [w604 w637 w695]
                          tunnel: [w604 w632 w692] -> w597
                          tunnel: [w603 w631 w691] -> w596
                          tunnel: w595 -> [w603 w621 _]
                          frame "check", Default {
                            n220 = local read "Red Stand"() -> (w610:bool)
                            n221 = local read "GO RED"() -> (w609:bool)
                            n222 = And(x=w610, y=w609) -> (x .and. y?=→"AND red":bool)
                            n223 = local read "Green Stand"() -> (w608:bool)
                            n224 = local read "GO GREEN"() -> (w611:bool)
                            n225 = And(x=w611, y=w608) -> (x .and. y?=w606:bool)
                            "AND green" <- w606
                            n226 = case shown="False" w606 {
                              tunnel: [w612 enum16{"check", "false", "true", "stop"}."true"] -> w605
                              frame False {
                                n227 = local read "AND red"() -> (w613:bool)
                                n228 = case shown="False" w613 {
                                tunnel: [enum16{"check", "false", "true", "stop"}."true" enum16{"check", "false", "true", "stop"}."false"] -> w612
                                frame True {
                                n229 = local write "Green True"(FALSE ("Green True")) -> ()
                                n230 = local write "Red True"(TRUE ("Red True")) -> ()
                                }
                                frame False {
                                }
                                }
                              }
                              frame True {
                                n231 = local write "Red True"(FALSE ("Red True")) -> ()
                                n232 = local write "Green True"(TRUE ("Green True")) -> ()
                              }
                            }
                          }
                          frame "false" {
                            n233 = flat-sequence {
                              tunnel: w637 -> [w642]
                              tunnel: [w641] -> w630
                              tunnel: [w640] -> w629
                              tunnel: w621 -> [w638]
                              tunnel: [w648] -> w636
                              tunnel: [w646] -> w635
                              tunnel: w630 -> [w649]
                              tunnel: w629 -> [w647]
                              tunnel: w636 -> [w655]
                              tunnel: w635 -> [w650]
                              tunnel: [w651] -> w625
                              tunnel: [w650] -> w623
                              tunnel: w625 -> [w657]
                              tunnel: [w662] -> w624
                              tunnel: w623 -> [w661]
                              tunnel: [w656] -> w622
                              tunnel: [w673] -> w634
                              tunnel: [w672] -> w633
                              tunnel: w624 -> [w670]
                              tunnel: w622 -> [w669]
                              tunnel: w634 -> [w677]
                              tunnel: w633 -> [w675]
                              tunnel: [w676] -> w628
                              tunnel: [w674] -> w627
                              tunnel: [w682] -> w632
                              tunnel: [w683] -> w631
                              tunnel: w628 -> [w683]
                              tunnel: w627 -> [w682]
                              tunnel: [enum16{"check", "false", "true", "stop"}."stop"] -> w626
                              frame #0 {
                                n234 = local read "Servo 2 (centering)"() -> (w639:u16)
                                n235 = xnode "Read/Write Control"("FPGA VI Reference In"=w638, "error in"=w642, "SERVO 2"=w639) -> ("FPGA VI Reference Out"=w641:refnum<k20>, "error out"=w640:errorcluster)
                              }
                              frame #1 {
                                n236 = call "sub_vi_gerakan_robot.vi"("error out"=w647, "Numeric"=u32 500, "steering frame velocity"=dbl[] [200.0, 0.0, 0.0], "FPGA VI Reference Out"=w649) -> ("error out 2"=w646:errorcluster, "STOP ?"=→"STOP ? 4":bool, "FPGA VI Reference Out 2"=w648:refnum<k20>)  [unwired: 5 in]
                              }
                              frame #2 {
                                n237 = call "line follow test.vi"("FPGA VI Reference Out"=w655, "steering frame velocity"=dbl[] [150.0, 0.0, 0.0], "Options"=enum16{"ke kiri", "ke kanan"}."ke kanan") -> ("FPGA VI Reference Out 2"=w651:refnum<k20>, "STOP ?"=→"STOP ? 5":bool)  [unwired: 6 in]
                              }
                              frame #3 {
                                n238 = local read "AND red"() -> (w659:bool)
                                n239 = case shown="False" w659 {
                                tunnel: [w663 w668] -> w658
                                frame False {
                                n240 = local read "Value diatas brp?"() -> (w664:u16)
                                n241 = To Unsigned Long Integer(number=w664) -> (unsigned 32bit integer=w663:u32)
                                }
                                frame True {
                                n242 = local read "Value diatas brp?"() -> (w667:u16)
                                n243 = local read "M5  DOWN TIMES PUT"() -> (w665:u32)
                                n244 = To Unsigned Long Integer(number=w667) -> (unsigned 32bit integer=w666:u32)
                                n245 = Subtract(x=w665, y=w666) -> (x-y=w668:u32)
                                }
                                }
                                n246 = call "M5 CONFIG.vi"("error in"=w661, "Enum"=enum16{"naik", "turun"}."turun", "berapa kali?"=w658, "FPGA VI Reference Out"=w657) -> ("error out"=w662:errorcluster, "FPGA VI Reference Out 2"=w656:refnum<k20>)  [unwired: 6 in]
                              }
                              frame #4 {
                                n247 = local read "Gripper Open"() -> (w671:u16)
                                n248 = xnode "Read/Write Control"("FPGA VI Reference In"=w669, "error in"=w670, "SERVO 3"=w671) -> ("FPGA VI Reference Out"=w673:refnum<k20>, "error out"=w672:errorcluster)
                              }
                              frame #5 {
                                n249 = call "sub_vi_gerakan_robot.vi"("error out"=w675, "Numeric"=u32 1000, "steering frame velocity"=dbl[] [0.0, -200.0, 0.0], "FPGA VI Reference Out"=w677) -> ("error out 2"=w674:errorcluster, "STOP ?"=→"STOP ? 6":bool, "FPGA VI Reference Out 2"=w676:refnum<k20>)  [unwired: 5 in]
                              }
                              frame #6 {
                              }
                            }
                          }
                          frame "true" {
                            n250 = flat-sequence {
                              tunnel: w695 -> [w698]
                              tunnel: [w700] -> w686
                              tunnel: [w699] -> w685
                              tunnel: [w702] -> w688
                              tunnel: [w701] -> w687
                              tunnel: w686 -> [w705]
                              tunnel: w685 -> [w704]
                              tunnel: [w712] -> w689
                              tunnel: w688 -> [w707]
                              tunnel: w687 -> [w710]
                              tunnel: [w706] -> w684
                              tunnel: [w722] -> w694
                              tunnel: [w721] -> w693
                              tunnel: w689 -> [w719]
                              tunnel: w684 -> [w718]
                              tunnel: w694 -> [w726]
                              tunnel: w693 -> [w724]
                              tunnel: [w725] -> w691
                              tunnel: [w723] -> w692
                              frame #0 {
                                n251 = call "sub_vi_gerakan_robot.vi"("error out"=w698, "Numeric"=u32 800, "steering frame velocity"=dbl[] [0.0, 150.0, 0.0]) -> ("error out 2"=w699:errorcluster, "FPGA VI Reference Out 2"=w700:refnum<k20>)  [unwired: 6 in, 1 out]
                              }
                              frame #1 {
                                n252 = local read "Servo 2 (centering)"() -> (w703:u16)
                                n253 = xnode "Read/Write Control"("FPGA VI Reference In"=w705, "error in"=w704, "SERVO 2"=w703) -> ("FPGA VI Reference Out"=w702:refnum<k20>, "error out"=w701:errorcluster)
                              }
                              frame #2 {
                                n254 = local read "AND green"() -> (w708:bool)
                                n255 = case shown="False" w708 {
                                tunnel: [u32 3 w715] -> w709
                                frame False {
                                }
                                frame True {
                                n256 = local read "Value diatas brp?"() -> (w716:u16)
                                n257 = To Unsigned Long Integer(number=w716) -> (unsigned 32bit integer=w717:u32)
                                n258 = Subtract(x=u32 3, y=w717) -> (x-y=w715:u32)
                                }
                                }
                                n259 = call "M5 CONFIG.vi"("error in"=w710, "Enum"=enum16{"naik", "turun"}."turun", "berapa kali?"=w709, "FPGA VI Reference Out"=w707) -> ("error out"=w712:errorcluster, "FPGA VI Reference Out 2"=w706:refnum<k20>)  [unwired: 6 in]
                              }
                              frame #3 {
                                n260 = local read "Gripper Open"() -> (w720:u16)
                                n261 = xnode "Read/Write Control"("FPGA VI Reference In"=w718, "error in"=w719, "SERVO 3"=w720) -> ("FPGA VI Reference Out"=w722:refnum<k20>, "error out"=w721:errorcluster)
                              }
                              frame #4 {
                                n262 = call "sub_vi_gerakan_robot.vi"("error out"=w724, "Numeric"=u32 1000, "steering frame velocity"=dbl[] [0.0, -150.0, 0.0], "FPGA VI Reference Out"=w726) -> ("error out 2"=w723:errorcluster, "STOP ?"=→"STOP ? 3":bool, "FPGA VI Reference Out 2"=w725:refnum<k20>)  [unwired: 5 in]
                              }
                            }
                          }
                        }
                        n263 = Equal?(x=w601, y=enum16{"check", "false", "true", "stop"}."stop") -> (x = y?=w599:bool)
                      }
                    }
                    frame #1 {
                    }
                  }
                }
                frame "room" {
                  n264 = local read "Green Stand"() -> (w740:bool)
                  n265 = local read "GO GREEN"() -> (w741:bool)
                  n266 = And(x=w740, y=w741) -> (x .and. y?=w737:bool)
                  n267 = local write "AND green"(w737) -> ()
                  n268 = local read "Red Stand"() -> (w738:bool)
                  n269 = local read "GO RED"() -> (w739:bool)
                  n270 = And(x=w738, y=w739) -> (x .and. y?=w736:bool)
                  n271 = case shown="True" w736 {
                    tunnel: [w742 T8."true"] -> w735
                    frame False {
                      n272 = local read "AND green"() -> (w743:bool)
                      n273 = case shown="True" w743 {
                        tunnel: [T8."false" T8."true"] -> w742
                        frame False {
                        }
                        frame True {
                          n274 = local read "Standcube diatas brp?"() -> (w746:u16)
                          n275 = Increment(x=w746) -> (x+1=w745:u16)
                          n276 = local write "Standcube diatas brp?"(w745) -> ()
                        }
                      }
                    }
                    frame True {
                    }
                  }
                }
                frame "true" {
                  n277 = flat-sequence {
                    tunnel: w763 -> [w768]
                    tunnel: [w767] -> w762
                    tunnel: [w766] -> w761
                    tunnel: w750 -> [w764]
                    tunnel: w762 -> [w772]
                    tunnel: w761 -> [w775]
                    tunnel: [w770] -> w753
                    tunnel: [w769] -> w752
                    tunnel: w753 -> [w776]
                    tunnel: w752 -> [w779]
                    tunnel: [w778] -> w751
                    tunnel: [w777] -> w749
                    tunnel: [w799] -> w760
                    tunnel: [w798] -> w759
                    tunnel: w751 -> [w796]
                    tunnel: w749 -> [w795]
                    tunnel: w760 -> [w804]
                    tunnel: w759 -> [w806]
                    tunnel: [w805] -> w758
                    tunnel: [w803] -> w757
                    tunnel: [w808] -> w754
                    tunnel: [w809] -> w755
                    tunnel: w758 -> [w809]
                    tunnel: w757 -> [w808]
                    tunnel: [T8."stop"] -> w756
                    frame #0 {
                      n278 = local read "Servo 2 (centering)"() -> (w765:u16)
                      n279 = xnode "Read/Write Control"("FPGA VI Reference In"=w764, "error in"=w768, "SERVO 2"=w765) -> ("FPGA VI Reference Out"=w767:refnum<k20>, "error out"=w766:errorcluster)
                    }
                    frame #1 {
                      n280 = call "sub_vi_gerakan_robot.vi"("error out"=w775, "Numeric"=u32 800, "steering frame velocity"=dbl[] [0.0, 150.0, 0.0], "FPGA VI Reference Out"=w772) -> ("error out 2"=w769:errorcluster, "STOP ?"=→"STOP ? 7":bool, "FPGA VI Reference Out 2"=w770:refnum<k20>)  [unwired: 5 in]
                    }
                    frame #2 {
                      n281 = disable-structure shown="Enabled" {
                        disable-tunnel: w779 -> [w786 w793]
                        disable-tunnel: [w785 w793] -> w778
                        disable-tunnel: [w781 w794] -> w777
                        disable-tunnel: w776 -> [w780 w794]
                        frame Disabled {
                          n282 = local read "AND green"() -> (w783:bool)
                          n283 = case shown="True" w783 {
                            tunnel: [w787 w792] -> w782
                            frame False {
                              n284 = local read "Value diatas brp?"() -> (w788:u16)
                              n285 = To Unsigned Long Integer(number=w788) -> (unsigned 32bit integer=w787:u32)
                            }
                            frame True {
                              n286 = local read "Value diatas brp?"() -> (w790:u16)
                              n287 = local read "M5  DOWN TIMES PUT"() -> (w791:u32)
                              n288 = To Unsigned Long Integer(number=w790) -> (unsigned 32bit integer=w789:u32)
                              n289 = Subtract(x=w791, y=w789) -> (x-y=w792:u32)
                            }
                          }
                          n290 = call "M5 CONFIG.vi"("error in"=w786, "Enum"=enum16{"naik", "turun"}."turun", "berapa kali?"=w782, "FPGA VI Reference Out"=w780) -> ("error out"=w785:errorcluster, "FPGA VI Reference Out 2"=w781:refnum<k20>)  [unwired: 6 in]
                        }
                        frame Enabled {
                        }
                      }
                    }
                    frame #3 {
                      n291 = local read "Gripper Open"() -> (w797:u16)
                      n292 = xnode "Read/Write Control"("FPGA VI Reference In"=w795, "error in"=w796, "SERVO 3"=w797) -> ("FPGA VI Reference Out"=w798:refnum<k20>, "error out"=w799:errorcluster)
                    }
                    frame #4 {
                      n293 = call "sub_vi_gerakan_robot.vi"("error out"=w804, "Numeric"=u32 800, "steering frame velocity"=dbl[] [0.0, -150.0, 0.0], "FPGA VI Reference Out"=w806) -> ("error out 2"=w803:errorcluster, "STOP ?"=→"STOP ? 8":bool, "FPGA VI Reference Out 2"=w805:refnum<k20>)  [unwired: 5 in]
                    }
                    frame #5 {
                    }
                  }
                }
                frame "false" {
                  n294 = flat-sequence {
                    tunnel: w825 -> [w827]
                    tunnel: [w828] -> w815
                    tunnel: [w827] -> w814
                    tunnel: [w833] -> w824
                    tunnel: [w832] -> w823
                    tunnel: w815 -> [w835]
                    tunnel: w814 -> [w834]
                    tunnel: w824 -> [w839]
                    tunnel: w823 -> [w842]
                    tunnel: [w837] -> w813
                    tunnel: [w836] -> w811
                    tunnel: w813 -> [w844]
                    tunnel: [w849] -> w812
                    tunnel: w811 -> [w848]
                    tunnel: [w843] -> w810
                    tunnel: [w860] -> w822
                    tunnel: [w859] -> w821
                    tunnel: w812 -> [w857]
                    tunnel: w810 -> [w856]
                    tunnel: w822 -> [w865]
                    tunnel: w821 -> [w867]
                    tunnel: [w866] -> w820
                    tunnel: [w864] -> w819
                    tunnel: [w869] -> w816
                    tunnel: [w870] -> w817
                    tunnel: w820 -> [w870]
                    tunnel: w819 -> [w869]
                    tunnel: [T8."stop"] -> w818
                    frame #0 {
                      n295 = call "line follow test.vi"("steering frame velocity"=dbl[] [150.0, 0.0, 0.0], "Options"=enum16{"ke kiri", "ke kanan"}."ke kanan") -> ("FPGA VI Reference Out 2"=w828:refnum<k20>, "STOP ?"=→"STOP ? 11":bool)  [unwired: 7 in]
                    }
                    frame #1 {
                      n296 = local read "Servo 2 (centering)"() -> (w831:u16)
                      n297 = xnode "Read/Write Control"("FPGA VI Reference In"=w835, "error in"=w834, "SERVO 2"=w831) -> ("FPGA VI Reference Out"=w833:refnum<k20>, "error out"=w832:errorcluster)
                    }
                    frame #2 {
                      n298 = call "sub_vi_gerakan_robot.vi"("error out"=w842, "Numeric"=u32 0, "steering frame velocity"=dbl[] [0.0, 0.0, 0.0], "FPGA VI Reference Out"=w839) -> ("error out 2"=w836:errorcluster, "STOP ?"=→"STOP ? 9":bool, "FPGA VI Reference Out 2"=w837:refnum<k20>)  [unwired: 5 in]
                    }
                    frame #3 {
                      n299 = local read "AND green"() -> (w845:bool)
                      n300 = case shown="True" w845 {
                        tunnel: [w850 w853] -> w846
                        frame False {
                          n301 = local read "M5  DOWN TIMES PUT"() -> (w851:u32)
                          n302 = To Unsigned Long Integer(number=w851) -> (unsigned 32bit integer=w850:u32)
                        }
                        frame True {
                          n303 = local read "Value diatas brp?"() -> (w855:u16)
                          n304 = local read "M5  DOWN TIMES PUT"() -> (w852:u32)
                          n305 = To Unsigned Long Integer(number=w855) -> (unsigned 32bit integer=w854:u32)
                          n306 = Subtract(x=w852, y=w854) -> (x-y=w853:u32)
                        }
                      }
                      n307 = call "M5 CONFIG.vi"("error in"=w848, "Enum"=enum16{"naik", "turun"}."turun", "berapa kali?"=w846, "FPGA VI Reference Out"=w844) -> ("error out"=w849:errorcluster, "FPGA VI Reference Out 2"=w843:refnum<k20>)  [unwired: 6 in]
                    }
                    frame #4 {
                      n308 = local read "Gripper Open"() -> (w858:u16)
                      n309 = xnode "Read/Write Control"("FPGA VI Reference In"=w856, "error in"=w857, "SERVO 3"=w858) -> ("FPGA VI Reference Out"=w859:refnum<k20>, "error out"=w860:errorcluster)
                    }
                    frame #5 {
                      n310 = call "sub_vi_gerakan_robot.vi"("error out"=w865, "Numeric"=u32 0, "steering frame velocity"=dbl[] [0.0, 0.0, 0.0], "FPGA VI Reference Out"=w867) -> ("error out 2"=w864:errorcluster, "STOP ?"=→"STOP ? 10":bool, "FPGA VI Reference Out 2"=w866:refnum<k20>)  [unwired: 5 in]
                    }
                    frame #6 {
                    }
                  }
                }
                frame "stop" {
                }
              }
              n311 = Equal?(x=w533, y=T8."stop") -> (x = y?=w535:bool)
            }
          }
        }
        n312 = case shown="0, Default" w475 {
          frame 1 {
            n313 = local write "Value diatas brp?"(u16 1 ("Value diatas brp?")) -> ()
          }
          frame 0, Default {
            n314 = local write "Value diatas brp?"(u16 0 ("Value diatas brp?")) -> ()
          }
        }
      }
      frame "GoNurse" {
        n315 = while {
          tunnel: [w879] -> w875
          tunnel: w877 -> [w879]
          tunnel: [w878] -> w874
          tunnel: w876 -> [w878]
          i -> [w884]
          stop <- w880 stop-if-true
          n316 = local read "total"() -> (w882:i16)
          n317 = local read "Index ke?"() -> (w889:i32)
          n318 = To Long Integer(number=w882) -> (32bit integer=w881:i32)
          n319 = local read "Go Nurse"() -> (w887:T4)
          n320 = local read "Output"() -> (w886:T4)
          n321 = Increment(x=w889) -> (x+1=w888:i32)
          n322 = Increment(x=w884) -> (x+1=w883:i32)
          n323 = Less Or Equal?(x=w881, y=w883) -> (x <= y?=w880:bool)
          n324 = Insert Into Array(array=w886, index=w888, new element=w887) -> (w885:T4)
          n325 = local write "Output"(w885) -> ()
        }
      }
      frame "Go1" {
        n326 = while {
          tunnel: [w895] -> w891
          tunnel: w893 -> [w895]
          tunnel: [w894] -> w890
          tunnel: w892 -> [w894]
          i -> [w900]
          stop <- w896 stop-if-true
          n327 = local read "total"() -> (w898:i16)
          n328 = local read "Index ke?"() -> (w905:i32)
          n329 = To Long Integer(number=w898) -> (32bit integer=w897:i32)
          n330 = local read "Go Room 1"() -> (w903:T4)
          n331 = local read "Output"() -> (w902:T4)
          n332 = Increment(x=w905) -> (x+1=w904:i32)
          n333 = Increment(x=w900) -> (x+1=w899:i32)
          n334 = Less Or Equal?(x=w897, y=w899) -> (x <= y?=w896:bool)
          n335 = Insert Into Array(array=w902, index=w904, new element=w903) -> (w901:T4)
          n336 = local write "Output"(w901) -> ()
        }
      }
      frame "Go2" {
        n337 = while {
          tunnel: [w911] -> w907
          tunnel: w909 -> [w911]
          tunnel: [w910] -> w906
          tunnel: w908 -> [w910]
          i -> [w916]
          stop <- w912 stop-if-true
          n338 = local read "total"() -> (w914:i16)
          n339 = local read "Index ke?"() -> (w921:i32)
          n340 = To Long Integer(number=w914) -> (32bit integer=w913:i32)
          n341 = local read "Go Room 2"() -> (w919:T4)
          n342 = local read "Output"() -> (w918:T4)
          n343 = Increment(x=w921) -> (x+1=w920:i32)
          n344 = Increment(x=w916) -> (x+1=w915:i32)
          n345 = Less Or Equal?(x=w913, y=w915) -> (x <= y?=w912:bool)
          n346 = Insert Into Array(array=w918, index=w920, new element=w919) -> (w917:T4)
          n347 = local write "Output"(w917) -> ()
        }
      }
    }
    n348 = Wait (ms)(milliseconds to wait=w42) -> ()  [unwired: 1 out]
    n349 = Increment(x=w49) -> (x+1=w54:i32)
    "Index ke?" <- w49
  }
  n350 = xnode "Close FPGA VI Reference"("FPGA VI Reference In"=w23, "error in"=w17) -> ("error out"=→"error out":errorcluster)
  "* times" <- 1.0 ("Numeric")
  "Green True" <- FALSE ("Green True")
  "Red True" <- FALSE ("Red True")
  "M5 down" <- i16 2500 ("M5 down")
  "M5 up" <- i16 3000 ("M5 up")
